vi "Configure NULL.vi"(7 "Target Trace (0: All)":i32(ring) items=["All", "Select"], 8 "error in (no error)":errorcluster, 9 "Status (0: ON)":i32(ring) items=["ON", "HOLD", "OFF"], 10 "Trace (0: U1)":i32(ring) items=["U1", "I1", "U2", "I2", "U3", "I3", "U4", "I4", "U5", "I5", "U6", "I6", "U All", "I All", "Speed", "Torque", "AUX1", "AUX2"], 11 "VISA resource name":refnum<visa-resource-name>) -> (0 "error out":errorcluster, 3 "VISA resource name out":refnum<visa-resource-name>)   [LabVIEW 2021, in "Yokogawa WT1800 Series.lvlib"]
doc: "Configures the NULL features.\nYou can use the NULL feature to subtract the DC offset while a measurement cable or external sensor is connected."
uses:
  <instrlib>/Yokogawa WT1800 Series/Yokogawa WT1800 Series.lvlib
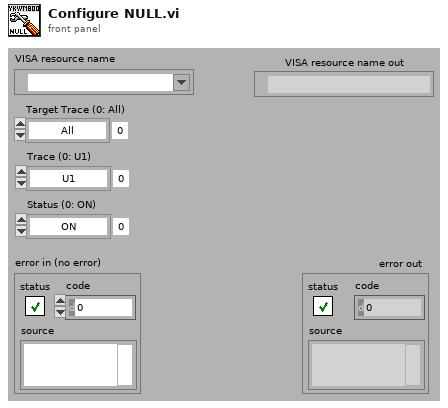
[diagram p1: front panel]
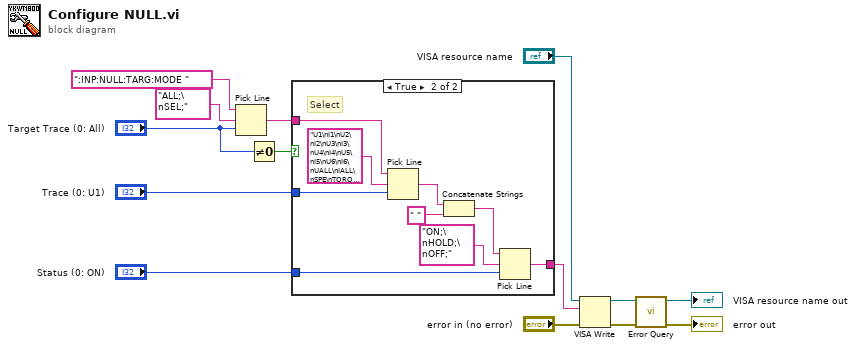
[diagram p0: block diagram]
diagram:
  n1 = Pick Line ("ライン選択")(string ("")=":INP:NULL:TARG:MODE " ("形式文字列"), multi-line string="ALL;\nSEL;" ("複数行文字列"), line index="Target Trace (0: All)") -> (output string=w6:string)
  n2 = Not Equal To 0?(x="Target Trace (0: All)") -> (x != 0?=w3:bool)
  n3 = case shown="True" w3 {
    tunnel: "Trace (0: U1)" -> [_ w23]
    tunnel: w6 -> [w15 w22]
    tunnel: "Status (0: ON)" -> [_ w18]
    tunnel: [w15 w16] -> w4
    frame False {
      # "All"
    }
    frame True {
      # "Select"
      n4 = Pick Line ("ライン選択")(string ("")=w22, multi-line string="U1\nI1\nU2\nI2\nU3\nI3\nU4\nI4\nU5\nI5\nU6\nI6\nUALL\nIALL\nSPE\nTORQ\nAUX1\nAUX2" ("複数行文字列"), line index=w23) -> (output string=w20:string)
      n5 = Concatenate Strings(w20, " " ("形式文字列")) -> (w17:string)
      n6 = Pick Line ("ライン選択")(string ("")=w17, multi-line string="ON;\nHOLD;\nOFF;" ("複数行文字列"), line index=w18) -> (output string=w16:string)
    }
  }
  n7 = VISA Write ("VISA書き込み")(VISA resource name="VISA resource name", write buffer=w4, error in (no error)="error in (no error)") -> (VISA resource name out=w14:refnum<visa-resource-name>, error out=w13:errorcluster)  [unwired: 1 out]
  n8 = call <instrlib>:"Error Query.vi"("error in (no error)"=w13, "VISA resource name"=w14) -> ("error out"=→"error out":errorcluster, "VISA resource name out"=→"VISA resource name out":refnum<visa-resource-name>)  [unwired: 6 in, 2 out]
